vi "NovaTech409A_PhaseToCommand_2DArray.vi"(1 "Novatech Phase [degrees]":dbl[][](array[numeric])) -> (0 "Novatech Command":u16[][](array[numeric]))   [LabVIEW 2013, in "Novatech 409A.lvlib"]
uses:
  Novatech 409A.lvlib
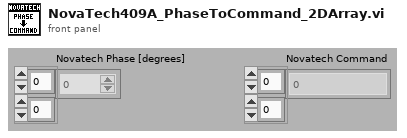
[diagram p1: front panel]
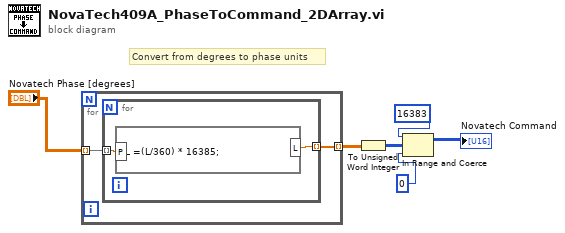
[diagram p0: block diagram]
diagram:
  # "Convert from degrees to phase units"
  n1 = for {
    tunnel: "Novatech Phase [degrees]" -> [w8] mode=indexing
    tunnel: [w7] -> w2 mode=indexing
    n2 = for {
      tunnel: w8 -> [w10] mode=indexing
      tunnel: [w9] -> w7 mode=indexing
      n3 = formula code="L =(L/360) * 16385;"("P"=w10) -> ("L"=w9:dbl)
    }
  }
  n4 = To Unsigned Word Integer(number=w2) -> (unsigned 16bit integer=w4:u16[][])
  n5 = In Range and Coerce(upper limit=u16 16383, x=w4, lower limit=u16 0) -> (coerced(x)=→"Novatech Command":u16[][])  [unwired: 1 out]
